vi "CMD_COS.vi"(8 "error in (no error)":errorcluster, 10 "Arguments":string[](array[string]), 11 "gScript Interpreter in":refnum<class "gScript Interpreter.lvclass">) -> (0 "error out":errorcluster, 3 "gScript Interpreter out":refnum<class "gScript Interpreter.lvclass">)   [LabVIEW 2017, in "gScript Interpreter.lvclass"]
uses:
  gScript Interpreter.lvclass
  Type Definitions/Memory Cell.ctl
  Type Definitions/Memory Cell Type Enum.ctl
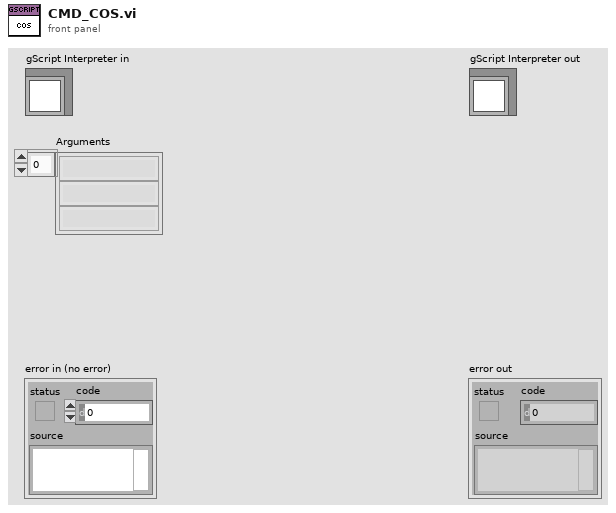
[diagram p1: front panel]
types:
  T1 = typedef "Memory Cell Type Enum.ctl" = enum16{"integer", "float", "vector", "rotation"}
  T2 = typedef "Memory Cell.ctl" = cluster{"type":T1, "x":dbl, "y":dbl, "z":dbl, "w":dbl}
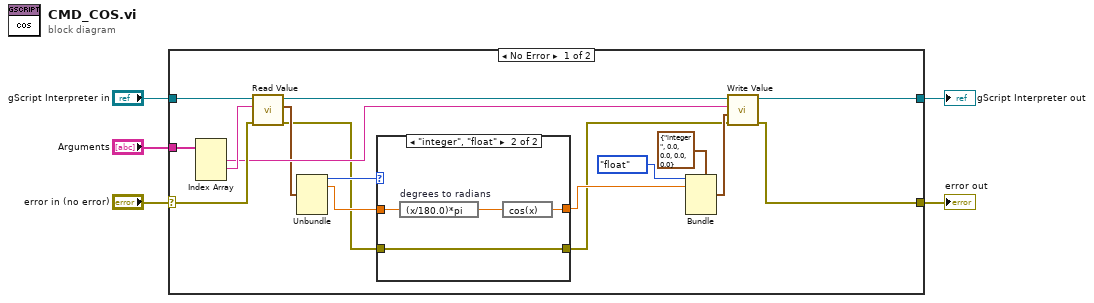
[diagram p0: block diagram]
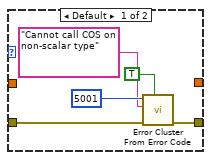
[diagram p2: hidden frame]
diagram:
  n1 = case shown="No Error" "error in (no error)" {
    selector: "error in (no error)" -> [w20 w33]
    tunnel: [w13 w33] -> w4
    tunnel: [w14 w32] -> w2
    tunnel: "gScript Interpreter in" -> [w21 w32]
    tunnel: "Arguments" -> [w22 _]
    frame No Error {
      n2 = Index Array(array=w22) -> (element #1=w18:string, element #2=w19:string)  [unwired: 3 in, 1 out]
      n3 = call-dynamic "Read Value.vi"("error in (no error)"=w20, "String in"=w19, "gScript Interpreter in"=w21) -> ("error out"=w7:errorcluster, "Memory Cell"=w17:T2, "gScript Interpreter out"=w12:refnum<class "gScript Interpreter.lvclass">)  [unwired: 6 in]
      n4 = Unbundle(w17) -> ("type"=w11:T1, "x"=w10:dbl)  [unwired: 3 out]
      n5 = case shown="\"integer\", \"float\"" w11 {
        tunnel: w10 -> [_ w29]
        tunnel: [_ w31] -> w9
        tunnel: w7 -> [w23 w30]
        tunnel: [w27 w30] -> w6
        frame Default {
          n6 = call <vilib>:"Error Cluster From Error Code.vi"("show call chain? (False)"=TRUE, "error in (no error)"=w23, "error message (\"\")"="Cannot call COS on non-scalar type" ("error message (\"\")"), "error code (0)"=5001) -> ("error out"=w27:errorcluster)  [unwired: 5 in]
        }
        frame "integer", "float" {
          n7 = expression code="(x/180.0)*pi" "degrees to radians"(w29) -> (w28:dbl)
          n8 = expression code="cos(x)"(w28) -> (w31:dbl)
        }
      }
      n9 = Bundle(cluster=T2 {"type"=enum."integer", "x"=0.0, "y"=0.0, "z"=0.0, "w"=0.0} ("Memory Cell"), "type"=Memory_Cell_Type_Enum."float", "x"=w9) -> (w15:T2)  [unwired: 3 in]
      n10 = call-dynamic "Write Value.vi"("error in (no error)"=w6, "Value"=w15, "Address"=w18, "gScript Interpreter in"=w12) -> ("error out"=w13:errorcluster, "gScript Interpreter out"=w14:refnum<class "gScript Interpreter.lvclass">)  [unwired: 6 in]
    }
    frame Error {
    }
  }
  "error out" <- w4
  "gScript Interpreter out" <- w2
